vi "SpreadsheetRead.vi"() -> ()   [LabVIEW 2015]
uses:
  <vilib>/Utility/file.llb/Write Delimited Spreadsheet (DBL).vi
panel:
  in  "Digitizing Parameters":T1
  in  "Waveform Parameters":T2
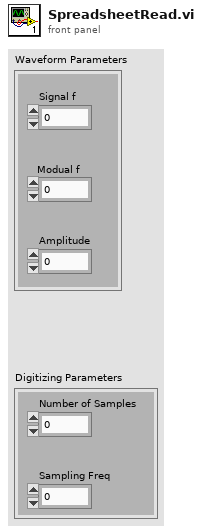
[diagram p1: front panel]
types:
  T1 = cluster{"Number of Samples":dbl, "Sampling Freq":dbl}
  T2 = cluster{"Signal f":dbl, "Modual f":dbl, "Amplitude":dbl}
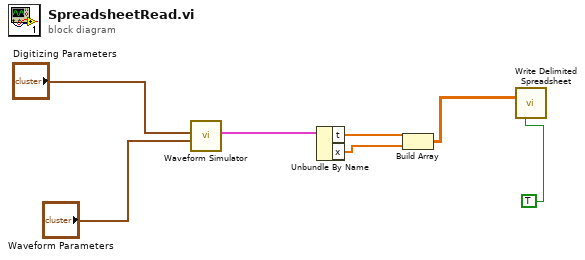
[diagram p0: block diagram]
diagram:
  n1 = call "Waveform Simulator.vi"("Waveform Parameters"="Waveform Parameters", "Digitizing Parameters"="Digitizing Parameters") -> ("output cluster"=w5:cluster{"t":dbl[], "x":dbl[]})  [unwired: 9 in]
  n2 = Unbundle By Name(w5) -> ("t"=w3:dbl[], "x"=w2:dbl[])
  n3 = Build Array(w3, w2) -> (w1:dbl[][])
  n4 = call-poly <vilib>:"Write Delimited Spreadsheet.vi"("2D data"=w1, "transpose? (F)"=TRUE) -> ()  [unwired: 12 in, 2 out]
